vi "ntr.flow-panel.set-element-2.vi"(4 "Enum 2":T1=enum."Out of Range", 8 "error in":errorcluster, 9 "Message Text":string, 10 "Boolean Text (empty: no change)":string, 11 "Ctl Refnum":refnum<vi>) -> (0 "error in":errorcluster)   [LabVIEW 2024]
uses:
  controls/type.nrt.elment-state.ctl
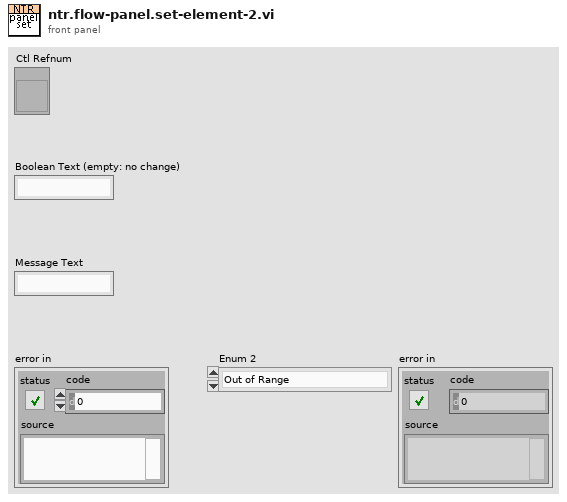
[diagram p1: front panel]
types:
  T1 = typedef "type.nrt.elment-state.ctl" = enum16{"No Change", "OFF", "In Range", "Out of Range", "Alarm"}
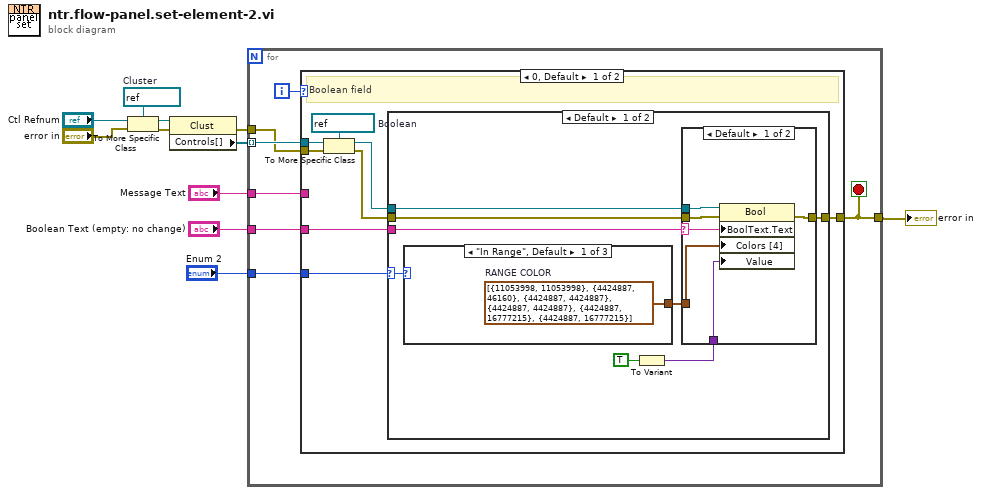
[diagram p0: block diagram]
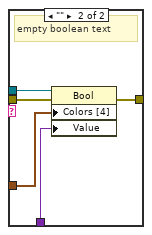
[diagram p2: hidden frame]
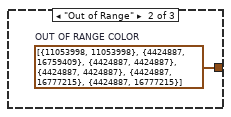
[diagram p3: hidden frame]
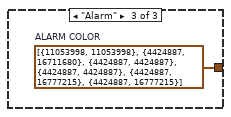
[diagram p4: hidden frame]
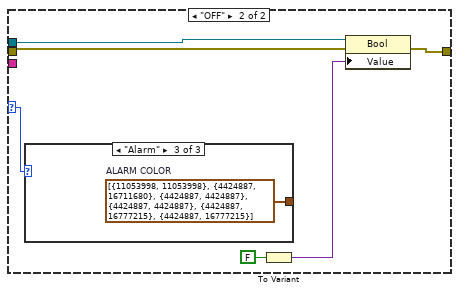
[diagram p5: hidden frame]
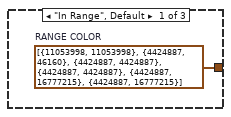
[diagram p6: hidden frame]
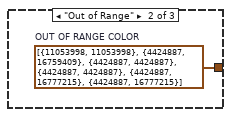
[diagram p7: hidden frame]
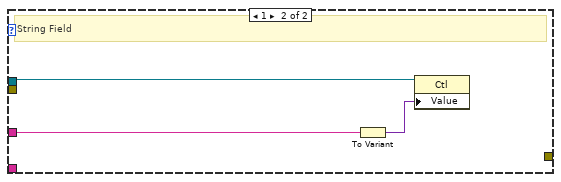
[diagram p8: hidden frame]
diagram:
  w5 = refnum<vi> refnum  # Cluster
  n1 = To More Specific Class(target class=w5, reference="Ctl Refnum", error in="error in") -> (specific class reference=w7:refnum<vi>, error out=w4:errorcluster)
  n2 = property class="Clust"(reference=w7, error in=w4) -> (error out=w3:errorcluster, "Controls[]"=w8:refnum<vi>[])  [unwired: 1 out]
  n3 = for {
    tunnel: w8 -> [w18] mode=indexing
    tunnel: "Boolean Text (empty: no change)" -> [w16]
    tunnel: "Enum 2" -> [w15]
    tunnel: "Message Text" -> [w14]
    tunnel: w3 -> [w13]
    tunnel: [w12] -> w2
    i -> [w17]
    stop <- w12 stop-if-true
    n4 = case shown="0, Default" w17 {
      tunnel: w18 -> [w26 w60]
      tunnel: w16 -> [w23 _]
      tunnel: w15 -> [w19 _]
      tunnel: w14 -> [_ w58]
      tunnel: w13 -> [w22 _]
      tunnel: [w20 _] -> w12
      frame 0, Default {
        w25 = refnum<vi> refnum  # Boolean
        # "Boolean field"
        n5 = To More Specific Class(target class=w25, reference=w26, error in=w22) -> (specific class reference=w24:refnum<vi>, error out=w21:errorcluster)
        n6 = case shown="Default" w19 {
          selector: w19 -> [w28 w49]
          tunnel: w24 -> [w33 w53]
          tunnel: w23 -> [w27 _]
          tunnel: w21 -> [w31 w52]
          tunnel: [w30 w51] -> w20
          frame Default {
            n7 = case shown="\"In Range\", Default" w28 {
              tunnel: [w46 w47 w48] -> w32
              frame "In Range", Default {
                w46 = cluster{u32, u32}[] [{11053998, 11053998}, {4424887, 46160}, {4424887, 4424887}, {4424887, 4424887}, {4424887, 16777215}, {4424887, 16777215}]  # RANGE COLOR
              }
              frame "Out of Range" {
                w47 = cluster{u32, u32}[] [{11053998, 11053998}, {4424887, 16759409}, {4424887, 4424887}, {4424887, 4424887}, {4424887, 16777215}, {4424887, 16777215}]  # OUT OF RANGE COLOR
              }
              frame "Alarm" {
                w48 = cluster{u32, u32}[] [{11053998, 11053998}, {4424887, 16711680}, {4424887, 4424887}, {4424887, 4424887}, {4424887, 16777215}, {4424887, 16777215}]  # ALARM COLOR
              }
            }
            n8 = To Variant(anything=TRUE) -> (Variant=w29:variant)
            n9 = case shown="Default" w27 {
              selector: w27 -> [w35 _]
              tunnel: w33 -> [w40 w45]
              tunnel: w32 -> [w39 w44]
              tunnel: w31 -> [w38 w43]
              tunnel: [w37 w42] -> w30
              tunnel: w29 -> [w36 w41]
              frame Default {
                n10 = property class="Bool"(reference=w40, error in=w38, "BoolText.Text"=w35, "Colors [4]"=w39, "Value"=w36) -> (error out=w37:errorcluster)  [unwired: 1 out]
              }
              frame "" {
                # "empty boolean text"
                n11 = property class="Bool"(reference=w45, error in=w43, "Colors [4]"=w44, "Value"=w41) -> (error out=w42:errorcluster)  [unwired: 1 out]
              }
            }
          }
          frame "OFF" {
            n12 = case shown="\"Alarm\"" w49 {
              tunnel: [w55 w56 w57] -> _
              frame "In Range", Default {
                w55 = cluster{u32, u32}[] [{11053998, 11053998}, {4424887, 46160}, {4424887, 4424887}, {4424887, 4424887}, {4424887, 16777215}, {4424887, 16777215}]  # RANGE COLOR
              }
              frame "Out of Range" {
                w56 = cluster{u32, u32}[] [{11053998, 11053998}, {4424887, 16759409}, {4424887, 4424887}, {4424887, 4424887}, {4424887, 16777215}, {4424887, 16777215}]  # OUT OF RANGE COLOR
              }
              frame "Alarm" {
                w57 = cluster{u32, u32}[] [{11053998, 11053998}, {4424887, 16711680}, {4424887, 4424887}, {4424887, 4424887}, {4424887, 16777215}, {4424887, 16777215}]  # ALARM COLOR
              }
            }
            n13 = To Variant(anything=FALSE) -> (Variant=w50:variant)
            n14 = property class="Bool"(reference=w53, error in=w52, "Value"=w50) -> (error out=w51:errorcluster)  [unwired: 1 out]
          }
        }
      }
      frame 1 {
        # "String Field"
        n15 = To Variant(anything=w58) -> (Variant=w59:variant)
        n16 = property class="Ctl"(reference=w60, "Value"=w59) -> ()  [unwired: 1 in, 2 out]
      }
    }
  }
  "error in" <- w2
